vi "niDTS BT Tx Test UTIL Merge DF1 and DF2.vi"(10 "DF Array":T1(array[cluster])) -> (2 "DF1 and DF2":T2)   [LabVIEW 2015, in "niDTS BT.lvlib"]
uses:
  niDTS BT.lvlib
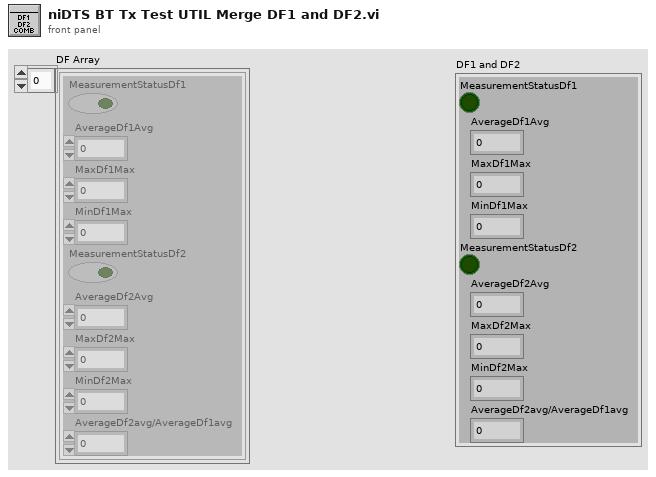
[diagram p1: front panel]
types:
  T1 = cluster{"MeasurementStatusDf1":bool, "AverageDf1Avg":dbl, "MaxDf1Max":dbl, "MinDf1Max":dbl, "MeasurementStatusDf2":bool, "AverageDf2Avg":dbl, "MaxDf2Max":dbl, "MinDf2Max":dbl, "AverageDf2avg/AverageDf1avg":dbl}[]
  T2 = cluster{"MeasurementStatusDf1":bool, "AverageDf1Avg":dbl, "MaxDf1Max":dbl, "MinDf1Max":dbl, "MeasurementStatusDf2":bool, "AverageDf2Avg":dbl, "MaxDf2Max":dbl, "MinDf2Max":dbl, "AverageDf2avg/AverageDf1avg":dbl}
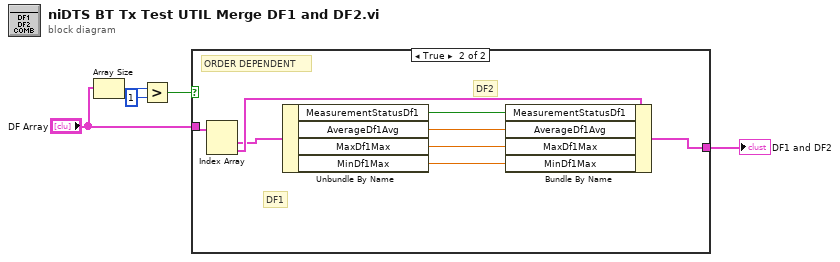
[diagram p0: block diagram]
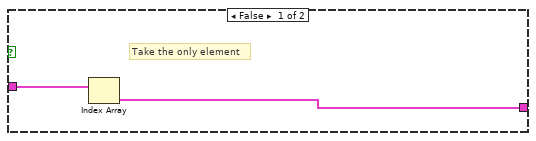
[diagram p2: hidden frame]
diagram:
  n1 = Array Size(array="DF Array") -> (size(s)=w5:i32)
  n2 = Greater?(x=w5, y=1) -> (0:w2:bool)
  n3 = case shown="True" w2 {
    tunnel: "DF Array" -> [w7 w11]
    tunnel: [w6 w8] -> w1
    frame False {
      # "Take the only element"
      n4 = Index Array(array=w7) -> (element=w6:T2)  [unwired: 1 in]
    }
    frame True {
      # "ORDER DEPENDENT"
      # "DF1"
      # "DF2"
      n5 = Index Array(array=w11) -> (element #1=w9:T2, element #2=w10:T2)  [unwired: 2 in]
      n6 = Unbundle By Name(w9) -> ("MeasurementStatusDf1"=w12:bool, "AverageDf1Avg"=w13:dbl, "MaxDf1Max"=w14:dbl, "MinDf1Max"=w15:dbl)
      n7 = Bundle By Name(cluster=w10, "MeasurementStatusDf1"=w12, "AverageDf1Avg"=w13, "MaxDf1Max"=w14, "MinDf1Max"=w15) -> (w8:T2)
    }
  }
  "DF1 and DF2" <- w1
